vi "AOTF_CreateAnalogPortsStepwise.vi"(0 "LineOnOff":bool[](array[boolean]), 7 "error in (no error)":errorcluster, 8 "AmplitudenNiveaus":dbl[](array[numeric])) -> (9 "LineOnOff[0]":bool, 11 "LineOnOff[1]":bool, 12 "task1":refnum<k21>, 13 "LineOnOff[2]":bool, 14 "#AmplitudenNiveaus":i32, 15 "LineOnOff[3]":bool, 16 "LineOnOff[7]":bool, 17 "LineOnOff[4]":bool, 18 "LineOnOff[6]":bool, 19 "LineOnOff[5]":bool, 20 "task2":refnum<k21>, 21 "task3":refnum<k21>, 22 "task4":refnum<k21>, 23 "task 5":refnum<k21>, 24 "task 6":refnum<k21>, 25 "task 8":refnum<k21>, 26 "task7":refnum<k21>, 27 "error out":errorcluster)   [LabVIEW 2011]
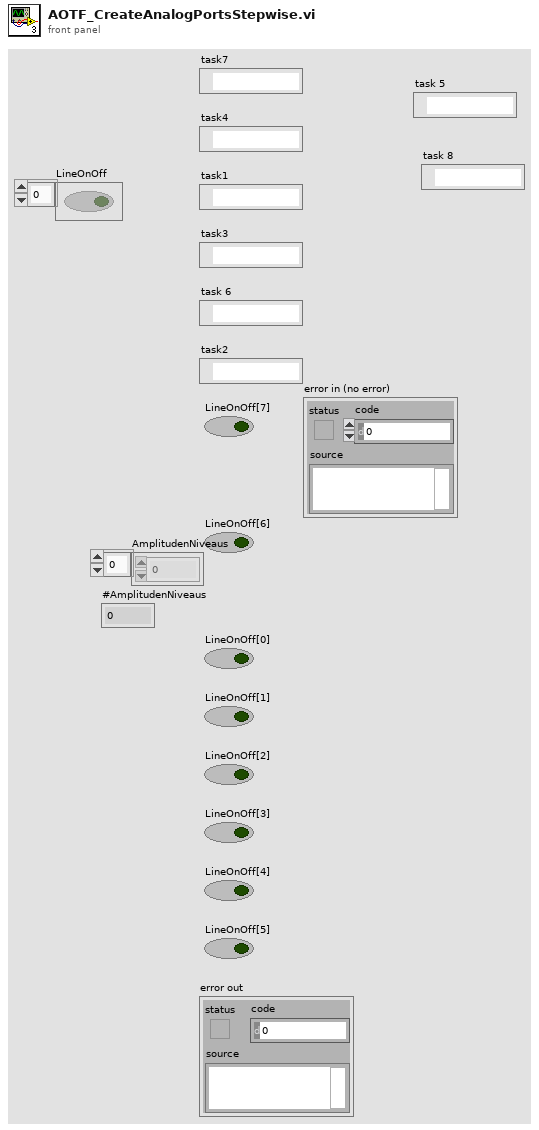
[diagram p1: front panel]
types:
  T1 = cluster{"LineOnOff[0]":bool, "LineOnOff[1]":bool, "LineOnOff[2]":bool, "LineOnOff[3]":bool, "LineOnOff[4]":bool, "LineOnOff[5]":bool, "LineOnOff[6]":bool, "LineOnOff[7]":bool, "LineOnOff[8]":bool}
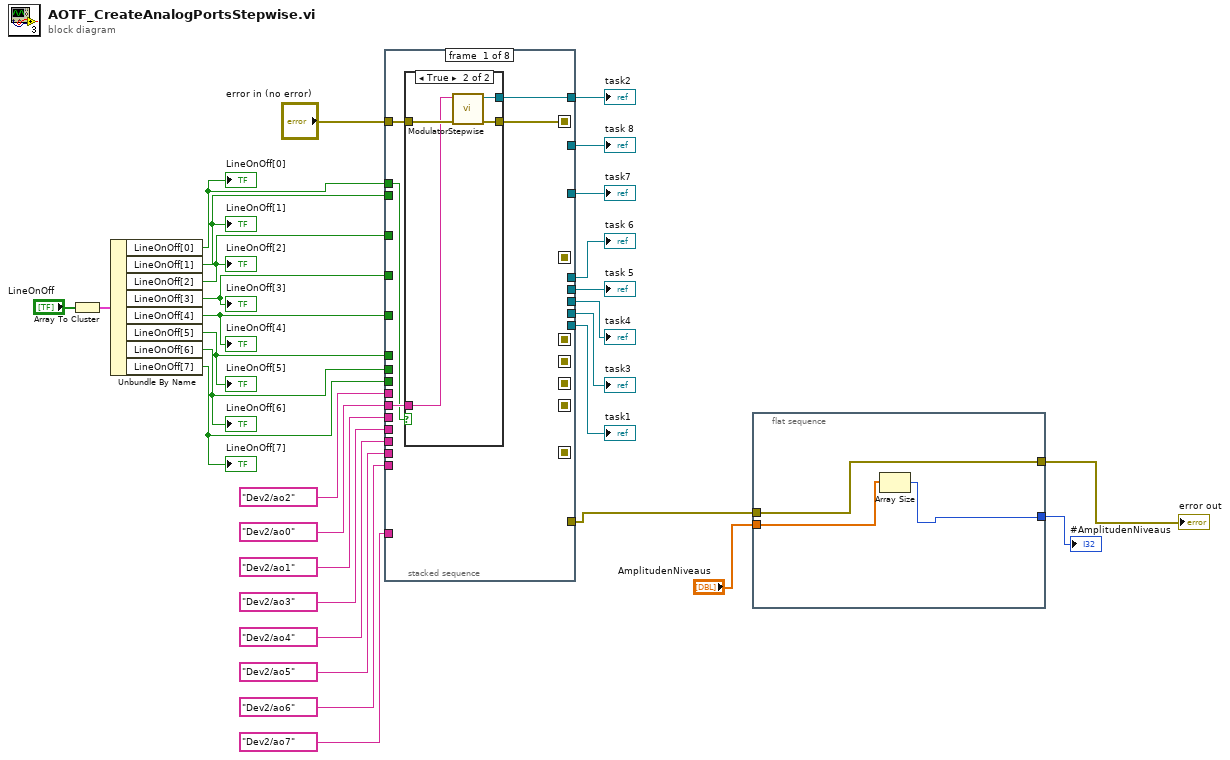
[diagram p0: block diagram]
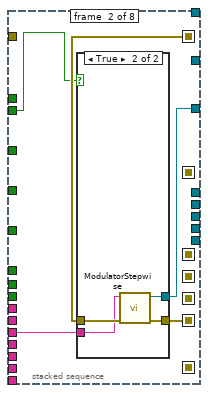
[diagram p3: hidden frame]
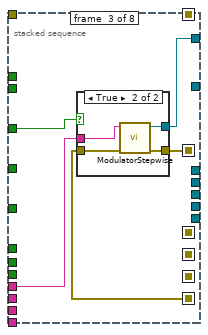
[diagram p5: hidden frame]
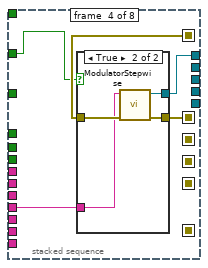
[diagram p7: hidden frame]
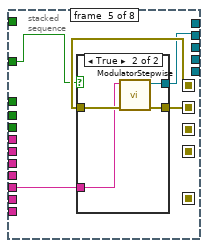
[diagram p9: hidden frame]
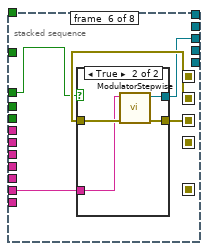
[diagram p11: hidden frame]
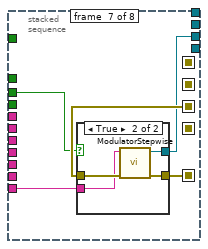
[diagram p13: hidden frame]
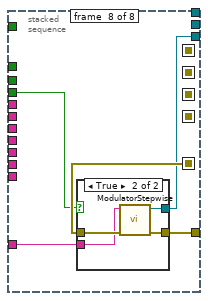
[diagram p15: hidden frame]
diagram:
  n1 = Array To Cluster(array="LineOnOff") -> (cluster=w14:T1)
  n2 = Unbundle By Name(w14) -> ("LineOnOff[0]"=w15:bool, "LineOnOff[1]"=w16:bool, "LineOnOff[2]"=w17:bool, "LineOnOff[3]"=w18:bool, "LineOnOff[4]"=w19:bool, "LineOnOff[5]"=w20:bool, "LineOnOff[6]"=w21:bool, "LineOnOff[7]"=w22:bool)
  "LineOnOff[7]" <- w22
  "LineOnOff[6]" <- w21
  "LineOnOff[5]" <- w20
  "LineOnOff[4]" <- w19
  "LineOnOff[3]" <- w18
  "LineOnOff[2]" <- w17
  "LineOnOff[1]" <- w16
  "LineOnOff[0]" <- w15
  n3 = stacked-sequence {
    seq-local: [w35 _ _ _ _ _ _ _] -> [_ w46 _ _ _ _ _ _]
    seq-local: [_ w45 _ _ _ _ _ _] -> [_ _ w56 _ _ _ _ _]
    seq-local: [_ _ w55 _ _ _ _ _] -> [_ _ _ w66 _ _ _ _]
    seq-local: [_ _ _ w65 _ _ _ _] -> [_ _ _ _ w76 _ _ _]
    seq-local: [_ _ _ _ w75 _ _ _] -> [_ _ _ _ _ w86 _ _]
    seq-local: [_ _ _ _ _ w85 _ _] -> [_ _ _ _ _ _ w96 _]
    seq-local: [_ _ _ _ _ _ w95 _] -> [_ _ _ _ _ _ _ w106]
    tunnel: "error in (no error)" -> [w36 _ _ _ _ _ _ _]
    tunnel: [_ _ _ _ _ _ _ w105] -> w3
    tunnel: tag "Dev2/ao0" ("physical channels") -> [w34 _ _ _ _ _ _ _]
    tunnel: tag "Dev2/ao1" ("physical channels") -> [_ w44 _ _ _ _ _ _]
    tunnel: tag "Dev2/ao2" ("physical channels") -> [_ _ w54 _ _ _ _ _]
    tunnel: tag "Dev2/ao3" ("physical channels") -> [_ _ _ w64 _ _ _ _]
    tunnel: tag "Dev2/ao4" ("physical channels") -> [_ _ _ _ w74 _ _ _]
    tunnel: tag "Dev2/ao5" ("physical channels") -> [_ _ _ _ _ w84 _ _]
    tunnel: tag "Dev2/ao6" ("physical channels") -> [_ _ _ _ _ _ w94 _]
    tunnel: tag "Dev2/ao7" ("physical channels") -> [_ _ _ _ _ _ _ w104]
    tunnel: w15 -> [w33 _ _ _ _ _ _ _]
    tunnel: w16 -> [_ w43 _ _ _ _ _ _]
    tunnel: w17 -> [_ _ w53 _ _ _ _ _]
    tunnel: w18 -> [_ _ _ w63 _ _ _ _]
    tunnel: w19 -> [_ _ _ _ w73 _ _ _]
    tunnel: w20 -> [_ _ _ _ _ w83 _ _]
    tunnel: w21 -> [_ _ _ _ _ _ w93 _]
    tunnel: w22 -> [_ _ _ _ _ _ _ w103]
    tunnel: [w32 _ _ _ _ _ _ _] -> w24
    tunnel: [_ w42 _ _ _ _ _ _] -> w25
    tunnel: [_ _ w52 _ _ _ _ _] -> w26
    tunnel: [_ _ _ w62 _ _ _ _] -> w27
    tunnel: [_ _ _ _ w72 _ _ _] -> w28
    tunnel: [_ _ _ _ _ w82 _ _] -> w29
    tunnel: [_ _ _ _ _ _ w92 _] -> w30
    tunnel: [_ _ _ _ _ _ _ w102] -> w31
    frame #0 {
      n4 = case shown="True" w33 {
        tunnel: w36 -> [w37 w39]
        tunnel: [w37 w41] -> w35
        tunnel: w34 -> [_ w38]
        tunnel: [_ w40] -> w32
        frame False {
        }
        frame True {
          n5 = call "ModulatorStepwise.vi"("error in (no error)"=w39, "physical channels"=w38) -> ("error out"=w41:errorcluster, "task out"=w40:refnum<k21>)  [unwired: 8 in]
        }
      }
    }
    frame #1 {
      n6 = case shown="True" w43 {
        tunnel: w46 -> [w47 w51]
        tunnel: [w47 w50] -> w45
        tunnel: w44 -> [_ w49]
        tunnel: [_ w48] -> w42
        frame False {
        }
        frame True {
          n7 = call "ModulatorStepwise.vi"("error in (no error)"=w51, "physical channels"=w49) -> ("error out"=w50:errorcluster, "task out"=w48:refnum<k21>)  [unwired: 8 in]
        }
      }
    }
    frame #2 {
      n8 = case shown="True" w53 {
        tunnel: w56 -> [w57 w60]
        tunnel: [w57 w61] -> w55
        tunnel: w54 -> [_ w58]
        tunnel: [_ w59] -> w52
        frame False {
        }
        frame True {
          n9 = call "ModulatorStepwise.vi"("error in (no error)"=w60, "physical channels"=w58) -> ("error out"=w61:errorcluster, "task out"=w59:refnum<k21>)  [unwired: 8 in]
        }
      }
    }
    frame #3 {
      n10 = case shown="True" w63 {
        tunnel: w66 -> [w67 w71]
        tunnel: [w67 w70] -> w65
        tunnel: w64 -> [_ w69]
        tunnel: [_ w68] -> w62
        frame False {
        }
        frame True {
          n11 = call "ModulatorStepwise.vi"("error in (no error)"=w71, "physical channels"=w69) -> ("error out"=w70:errorcluster, "task out"=w68:refnum<k21>)  [unwired: 8 in]
        }
      }
    }
    frame #4 {
      n12 = case shown="True" w73 {
        tunnel: w76 -> [w77 w80]
        tunnel: [w77 w81] -> w75
        tunnel: w74 -> [_ w78]
        tunnel: [_ w79] -> w72
        frame False {
        }
        frame True {
          n13 = call "ModulatorStepwise.vi"("error in (no error)"=w80, "physical channels"=w78) -> ("error out"=w81:errorcluster, "task out"=w79:refnum<k21>)  [unwired: 8 in]
        }
      }
    }
    frame #5 {
      n14 = case shown="True" w83 {
        tunnel: w86 -> [w87 w90]
        tunnel: [w87 w91] -> w85
        tunnel: w84 -> [_ w89]
        tunnel: [_ w88] -> w82
        frame False {
        }
        frame True {
          n15 = call "ModulatorStepwise.vi"("error in (no error)"=w90, "physical channels"=w89) -> ("error out"=w91:errorcluster, "task out"=w88:refnum<k21>)  [unwired: 8 in]
        }
      }
    }
    frame #6 {
      n16 = case shown="True" w93 {
        tunnel: w96 -> [w97 w101]
        tunnel: [w97 w100] -> w95
        tunnel: w94 -> [_ w99]
        tunnel: [_ w98] -> w92
        frame False {
        }
        frame True {
          n17 = call "ModulatorStepwise.vi"("error in (no error)"=w101, "physical channels"=w99) -> ("error out"=w100:errorcluster, "task out"=w98:refnum<k21>)  [unwired: 8 in]
        }
      }
    }
    frame #7 {
      n18 = case shown="True" w103 {
        tunnel: w106 -> [w107 w111]
        tunnel: [w107 w110] -> w105
        tunnel: w104 -> [_ w109]
        tunnel: [_ w108] -> w102
        frame False {
        }
        frame True {
          n19 = call "ModulatorStepwise.vi"("error in (no error)"=w111, "physical channels"=w109) -> ("error out"=w110:errorcluster, "task out"=w108:refnum<k21>)  [unwired: 8 in]
        }
      }
    }
  }
  "task1" <- w31
  "task3" <- w30
  "task4" <- w29
  "task 5" <- w28
  "task 6" <- w27
  "task 8" <- w26
  "task7" <- w25
  "task2" <- w24
  n20 = flat-sequence {
    tunnel: [w114] -> w4
    tunnel: w3 -> [w114]
    tunnel: [w113] -> w2
    tunnel: "AmplitudenNiveaus" -> [w112]
    frame #0 {
      n21 = Array Size(array=w112) -> (size(s)=w113:i32)
    }
  }
  "error out" <- w4
  "#AmplitudenNiveaus" <- w2
